vi "Zeros to Polynomial.vi"(1 "Zeros":cdb[](array[numeric]) format="%.2f") -> (0 "Polynomial":cdb[](array[numeric]) format="%.2f")   [LabVIEW 2017, in "NI_AdvCtrl_continuous linear.lvlib"]
doc: "LabVIEW no longer supports this VI. You can obtain similar functionality by installing the LabVIEW Simulation Module."
uses:
  <vilib>/addons/control/advanced/NI_AdvCtrl_continuous linear.lvlib
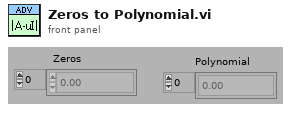
[diagram p1: front panel]
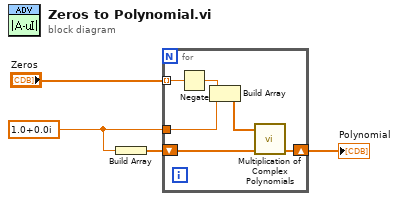
[diagram p0: block diagram]
diagram:
  w3 = cdb 1.0+0.0i
  n1 = Build Array(w3) -> (w1:cdb[])
  n2 = for {
    tunnel: "Zeros" -> [w10] mode=indexing
    shift-right: [w8] -> w4
    shift-left: w1 -> [w9]
    tunnel: w3 -> [w5]
    n3 = Negate(x=w10) -> (-x=w6:cdb)
    n4 = Build Array(w6, w5) -> (w7:cdb[])
    n5 = call <vilib>:"Multiplication of Complex Polynomials.vi"("Q"=w9, "P"=w7) -> ("P*Q"=w8:cdb[])
  }
  "Polynomial" <- w4
